vi "Polytec.vi"(0 "RS232":refnum<visa-resource-name>="ASRL27::INSTR", 2 "Strings":string[](array[string])) -> (7 "RS232 out":refnum<visa-resource-name>="ASRL27::INSTR", 9 "String Read":string)   [LabVIEW 2022 SP3]
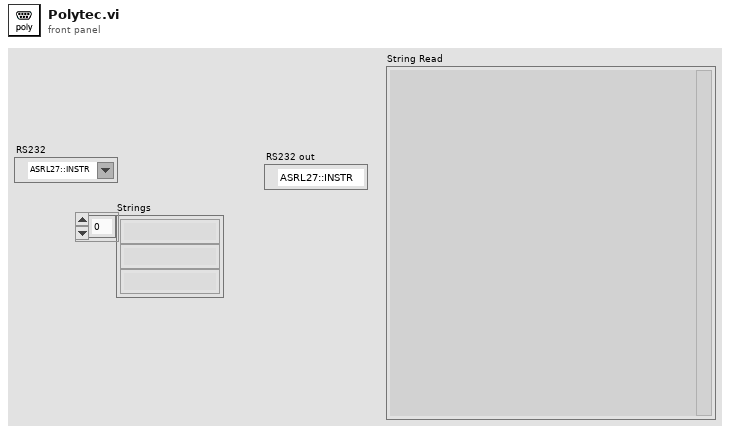
[diagram p1: front panel]
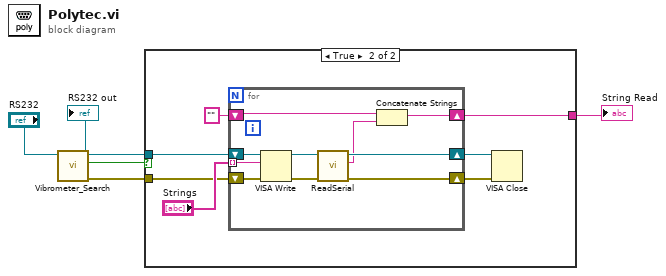
[diagram p0: block diagram]
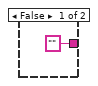
[diagram p2: hidden frame]
diagram:
  n1 = call "Vibrometer_Search.vi"("VISA Refnum in"="RS232") -> ("error out"=w4:errorcluster, "Success?"=w1:bool, "VISA Refnum out"=w3:refnum<visa-resource-name>)  [unwired: 8 in]
  "RS232 out" <- w3
  n2 = case shown="True" w1 {
    tunnel: w4 -> [_ w9]
    tunnel: w3 -> [_ w8]
    tunnel: ["" ("String Read") w7] -> w2
    frame False {
    }
    frame True {
      n3 = for {
        shift-right: [w23] -> w13
        shift-left: w9 -> [w21]
        shift-right: [w22] -> w12
        shift-left: w8 -> [w18]
        tunnel: "Strings" -> [w17] mode=indexing
        shift-right: [w14] -> w7
        shift-left: "" ("String Read") -> [w16]
        n4 = VISA Write(VISA resource name=w18, write buffer=w17, error in (no error)=w21) -> (VISA resource name out=w20:refnum<visa-resource-name>, error out=w19:errorcluster)  [unwired: 1 out]
        n5 = call "ReadSerial.vi"("error in (no error)"=w19, "VISA Refnum in"=w20) -> ("error out"=w23:errorcluster, "String Read"=w15:string, "VISA Refnum out"=w22:refnum<visa-resource-name>)  [unwired: 7 in]
        n6 = Concatenate Strings(w16, w15) -> (w14:string)
      }
      n7 = VISA Close(VISA resource name=w12, error in (no error)=w13) -> ()  [unwired: 1 out]
    }
  }
  "String Read" <- w2
